vi "Motor-Maker-Triangle RD.vi"() -> ()   [LabVIEW 2021]
panel:
  in  "X Volta":dbl
  out "Motor X\nLigado volt 3":bool=TRUE
  in  "Subida X Descida Y n vezes":i32
  out "Motor Y\nLigado ida 2":bool=TRUE
  in  "Y Descida 2":dbl
  out "Motor X\nLigado ida 2":bool=TRUE
  in  "Xsubida 2":dbl
  in  "SubidaXY em numero par":i32
  in  "Ysubida":dbl
  out "Motor Y\nLigado ida":bool=TRUE
  in  "Xsubida":dbl
  out "Motor X\nLigado ida":bool=TRUE
  # "numero do for loop"
  # "numero do for loop"
  # "N. do motor"
  # "N. do motor"
  # "N. da volta do x"
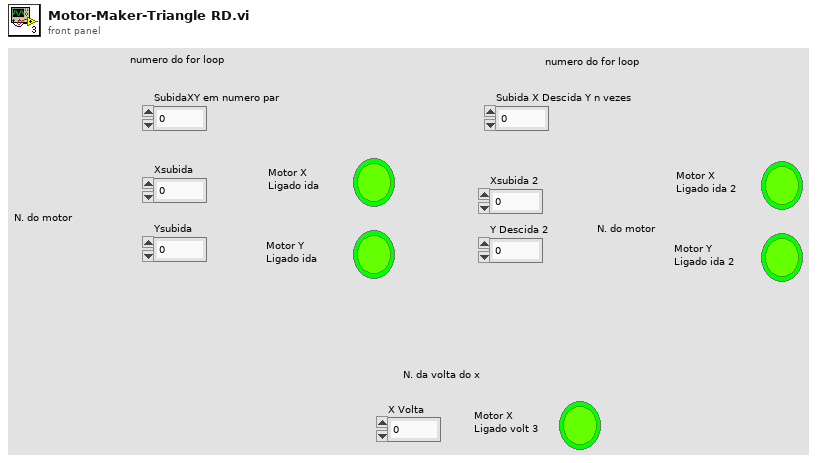
[diagram p1: front panel]
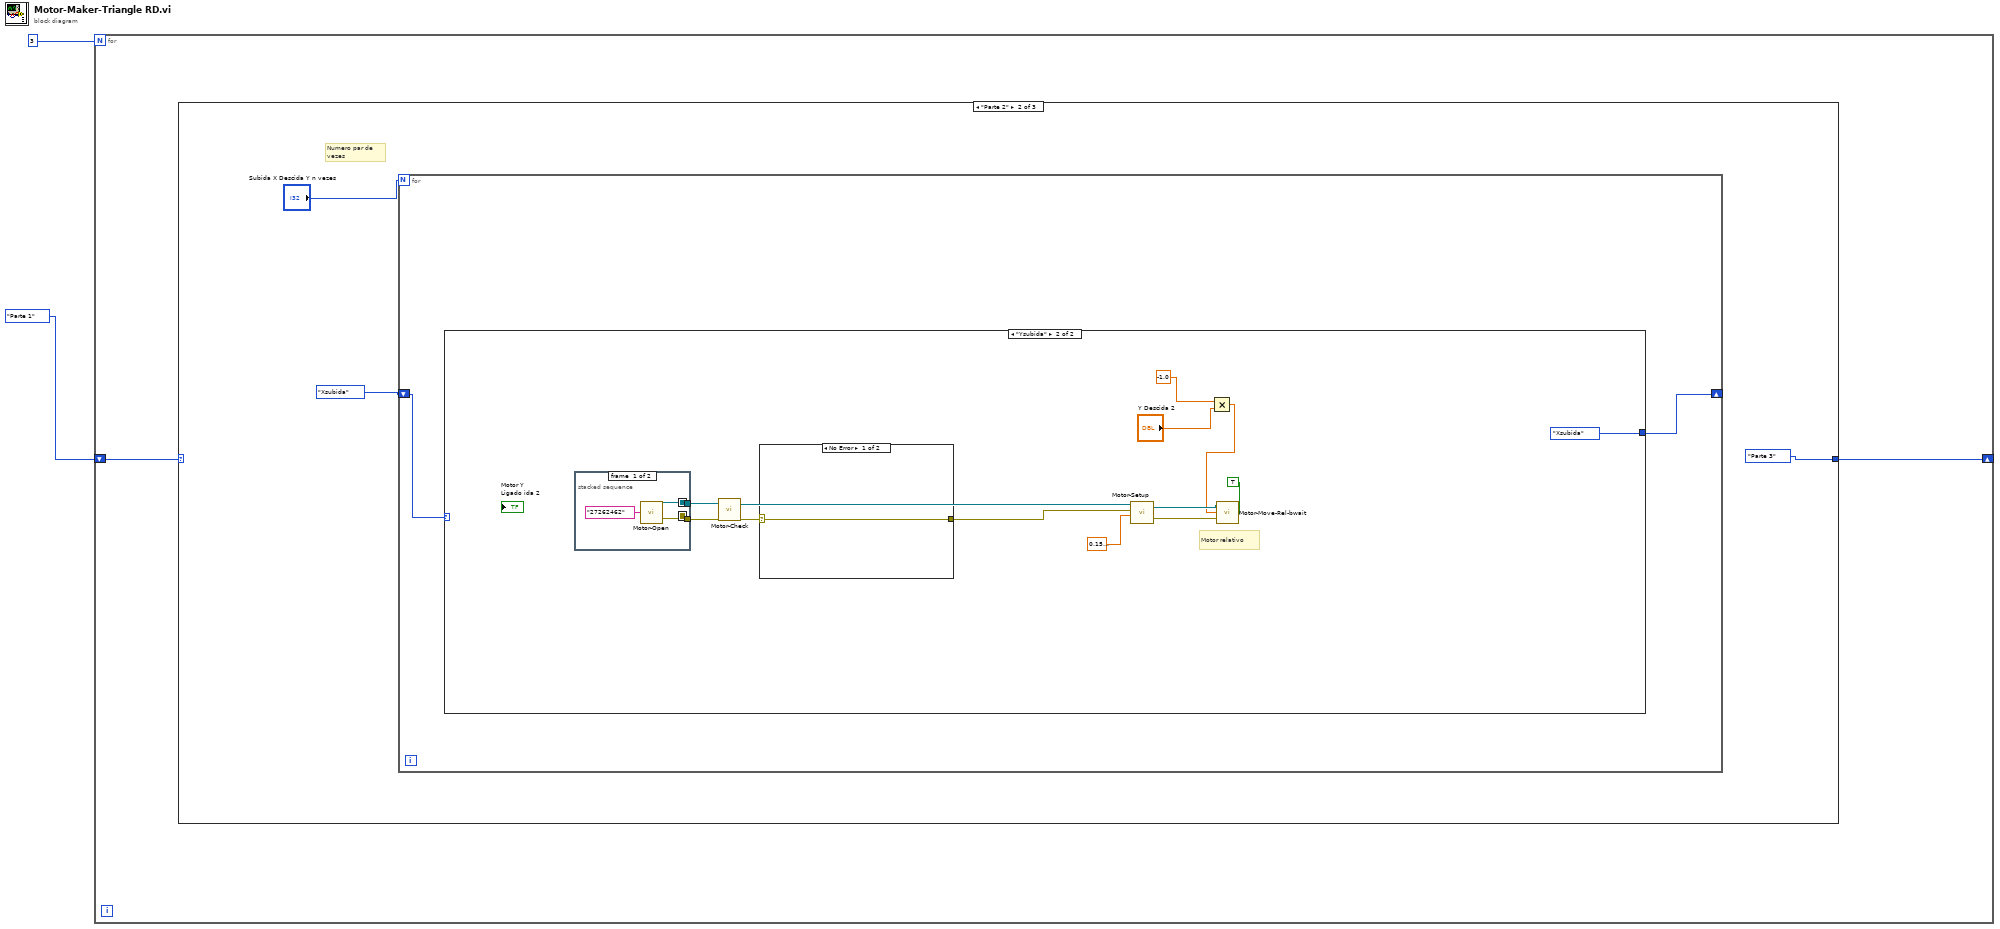
[diagram p0: block diagram]
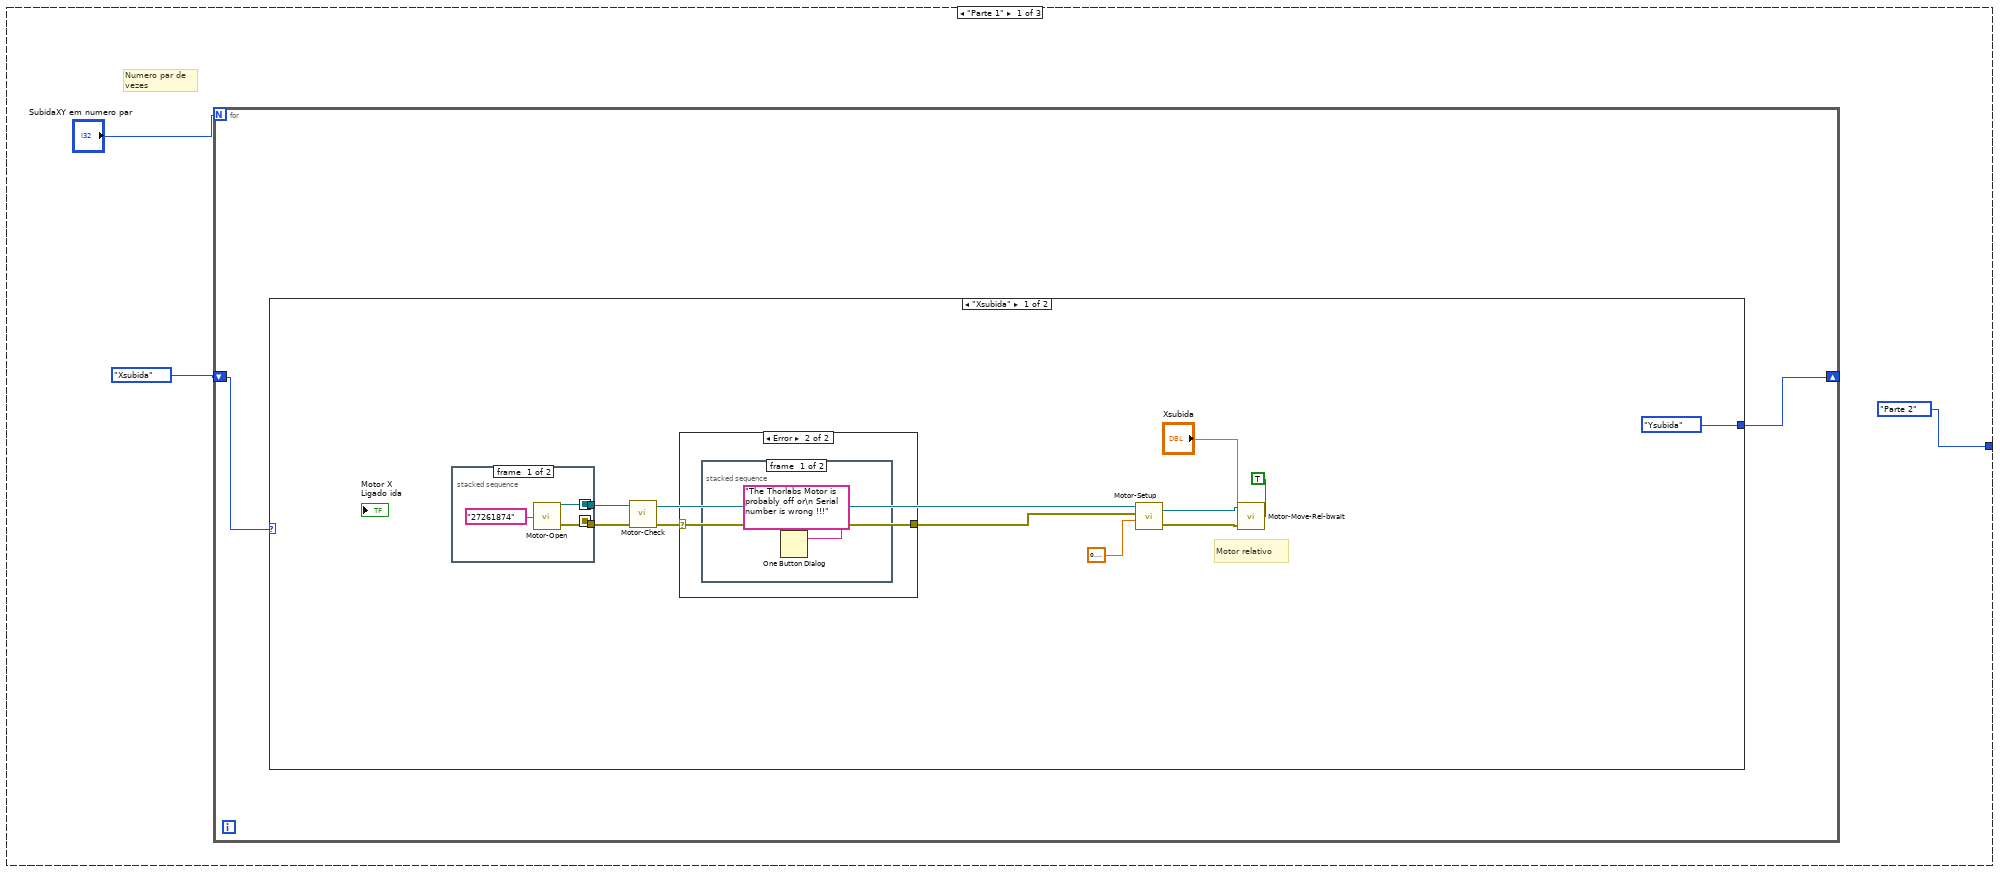
[diagram p2: hidden frame]
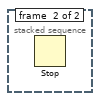
[diagram p4: hidden frame]
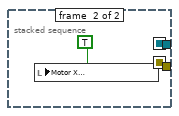
[diagram p5: hidden frame]
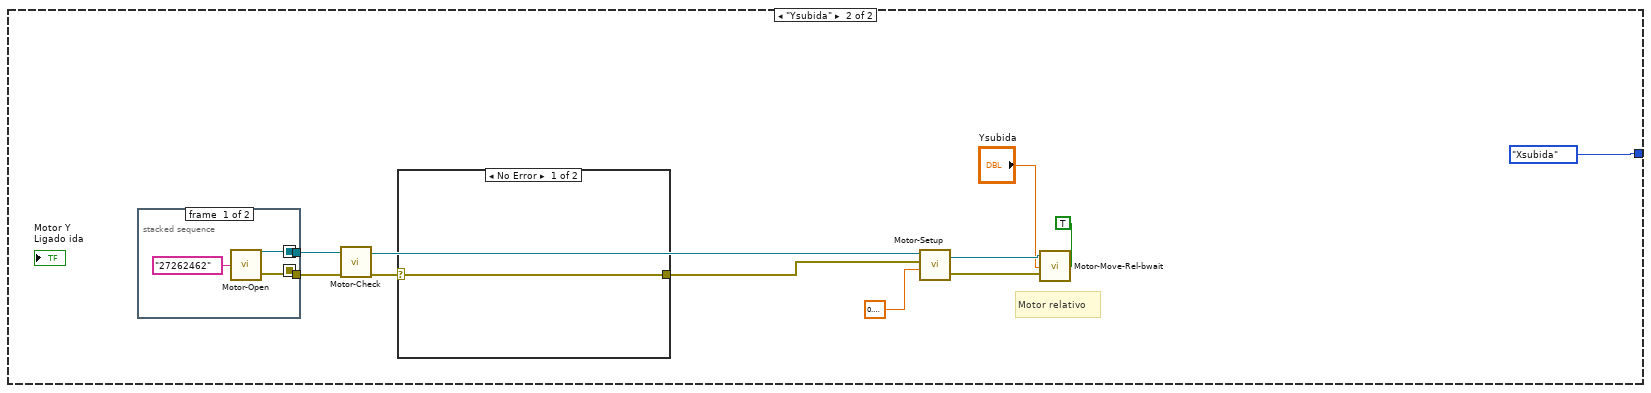
[diagram p6: hidden frame]
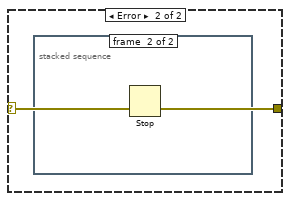
[diagram p7: hidden frame]
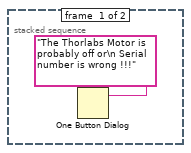
[diagram p8: hidden frame]
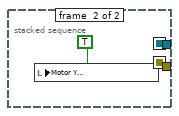
[diagram p9: hidden frame]
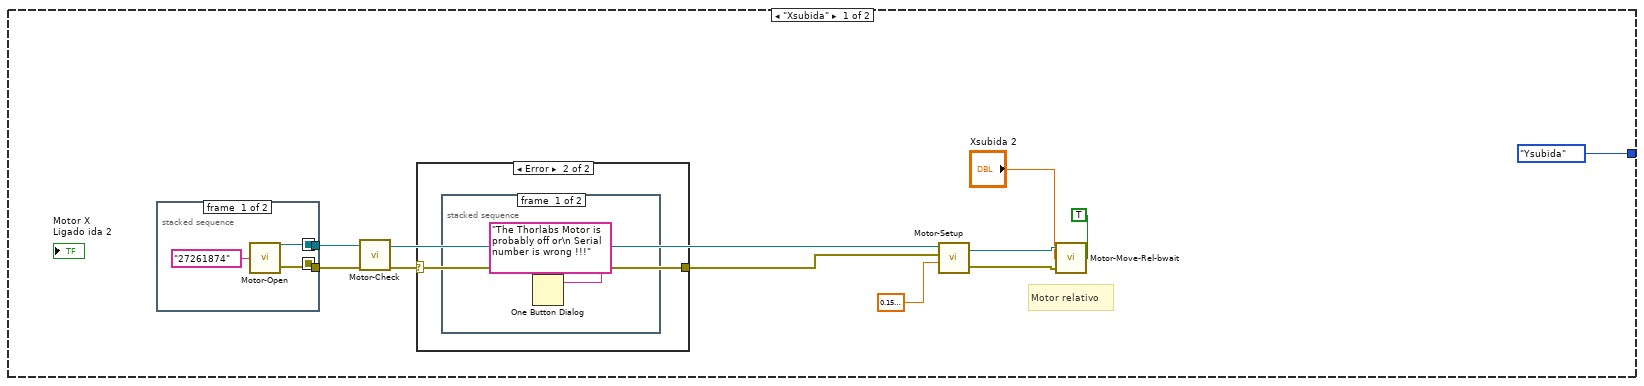
[diagram p10: hidden frame]
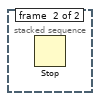
[diagram p12: hidden frame]
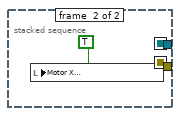
[diagram p13: hidden frame]
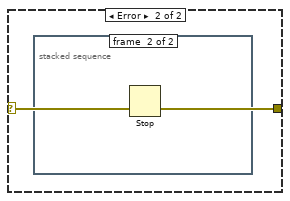
[diagram p14: hidden frame]
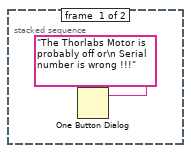
[diagram p15: hidden frame]
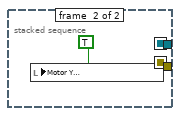
[diagram p16: hidden frame]
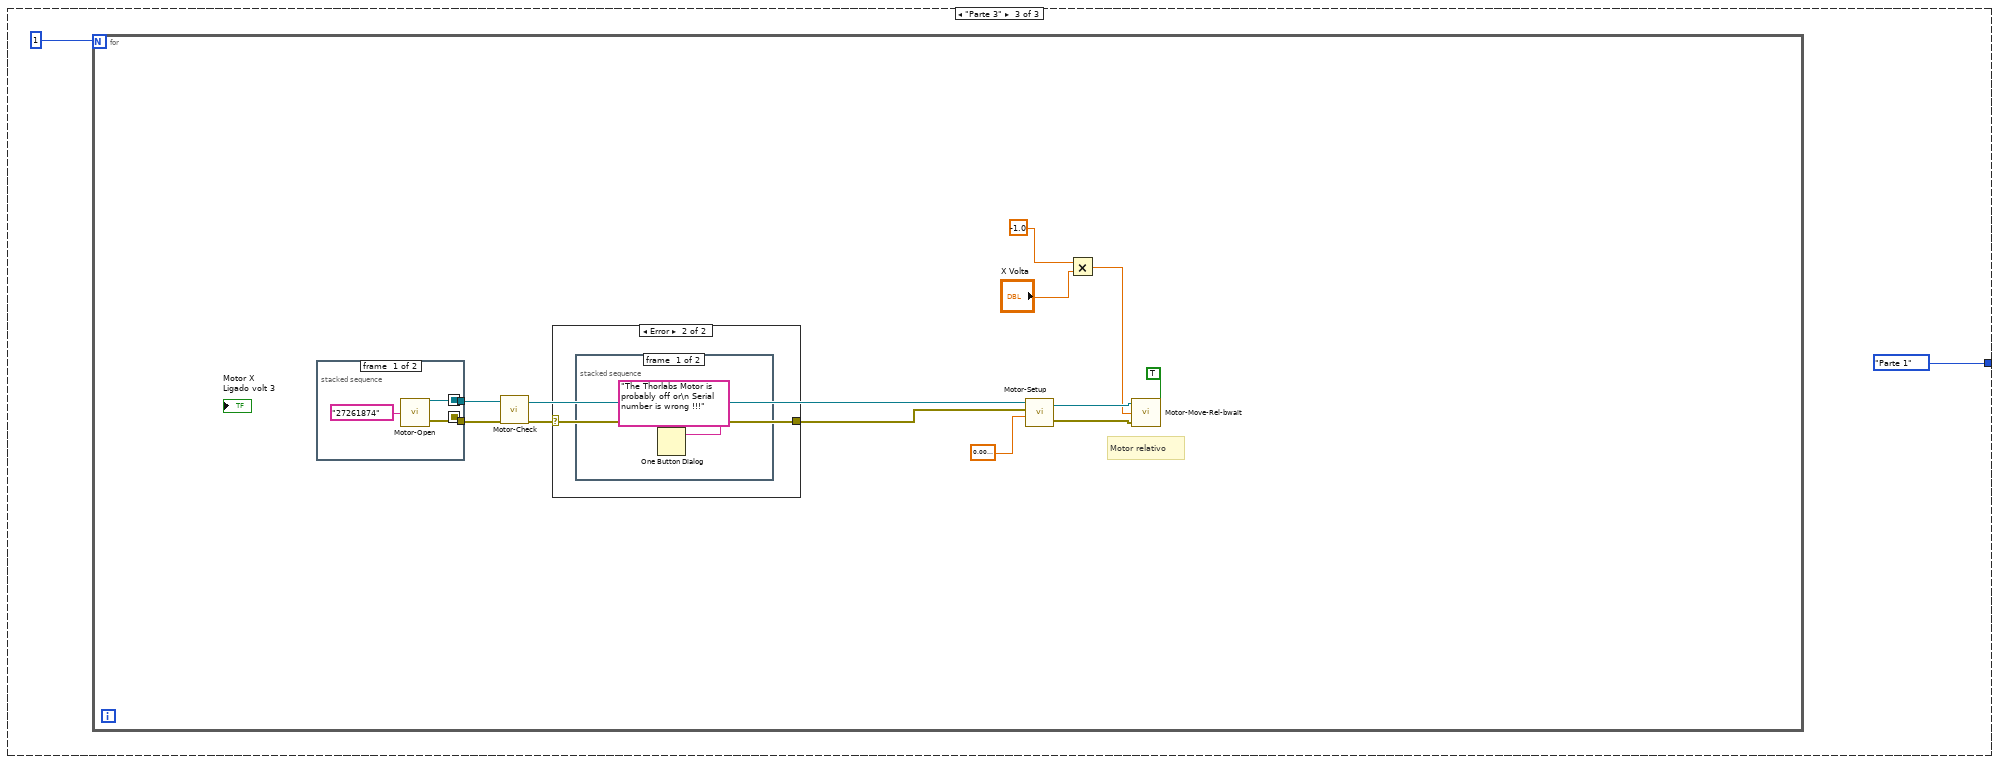
[diagram p17: hidden frame]
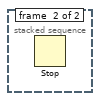
[diagram p19: hidden frame]
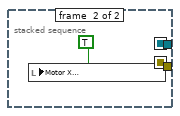
[diagram p20: hidden frame]
diagram:
  n1 = for {
    N: 3 -> [_]
    shift-right: [w3] -> _
    shift-left: enum16{"Parte 1", "Parte 2", "Parte 3"}."Parte 1" -> [w4]
    n2 = case shown="\"Parte 2\"" w4 {
      tunnel: [enum16{"Parte 1", "Parte 2", "Parte 3"}."Parte 2" enum16{"Parte 1", "Parte 2", "Parte 3"}."Parte 3" enum16{"Parte 1", "Parte 2", "Parte 3"}."Parte 1"] -> w3
      frame "Parte 1" {
        # "Numero par de vezes"
        n3 = for {
          N: "SubidaXY em numero par" -> [_]
          shift-right: [w8] -> _
          shift-left: enum16{"Xsubida", "Ysubida"}."Xsubida" -> [w9]
          n4 = case shown="\"Xsubida\"" w9 {
            tunnel: [enum16{"Xsubida", "Ysubida"}."Ysubida" enum16{"Xsubida", "Ysubida"}."Xsubida"] -> w8
            frame "Xsubida" {
              # "Motor relativo"
              n5 = stacked-sequence {
                seq-local: [w26 _] -> [_ w29]
                seq-local: [w25 _] -> [_ w28]
                tunnel: [_ w29] -> w20
                tunnel: [_ w28] -> w19
                frame #0 {
                  n6 = call "Motor-Open.vi"("S/N Motor"="27261874") -> ("MG17Motor 2"=w26:refnum<k7>, "error out"=w25:errorcluster)
                }
                frame #1 {
                  n7 = local write "Motor X\nLigado ida"(TRUE ("Motor3\nLigado")) -> ()
                }
              }
              n8 = call "Motor-Check.vi"("error in (no error)"=w19, "Automation Refnum in"=w20) -> ("error out"=w18:errorcluster, "Automation Refnum out"=w17:refnum<k7>)  [unwired: 8 in]
              n9 = case shown="Error" w18 {
                selector: w18 -> [w21 w22]
                tunnel: [w21 w22] -> w16
                frame No Error {
                }
                frame Error {
                  n10 = stacked-sequence {
                    frame #0 {
                      n11 = One Button Dialog(message="The Thorlabs Motor is probably off or\n Serial number is wrong !!!") -> ()  [unwired: 1 in, 1 out]
                    }
                    frame #1 {
                      n12 = Stop() -> ()  [unwired: 1 in]
                    }
                  }
                }
              }
              n13 = call "Motor-Setup.vi"("Velocidade"=sgl 0.1, "error"=w16, "MG17Motor A"=w17) -> ("error out"=w11:errorcluster, "MG17Motor out"=w12:refnum<k7>)  [unwired: 1 in]
              n14 = call "Motor-Move-Rel-bwait.vi"("bWait"=TRUE, "error"=w11, "Posição"="Xsubida", "MG17Motor A"=w12) -> ()  [unwired: 2 out]
            }
            frame "Ysubida" {
              # "Motor relativo"
              n15 = stacked-sequence {
                seq-local: [w46 _] -> [_ w49]
                seq-local: [w45 _] -> [_ w48]
                tunnel: [_ w49] -> w40
                tunnel: [_ w48] -> w39
                frame #0 {
                  n16 = call "Motor-Open.vi"("S/N Motor"="27262462") -> ("MG17Motor 2"=w46:refnum<k7>, "error out"=w45:errorcluster)
                }
                frame #1 {
                  n17 = local write "Motor Y\nLigado ida"(TRUE ("Motor3\nLigado")) -> ()
                }
              }
              n18 = call "Motor-Check.vi"("error in (no error)"=w39, "Automation Refnum in"=w40) -> ("error out"=w38:errorcluster, "Automation Refnum out"=w37:refnum<k7>)  [unwired: 8 in]
              n19 = case shown="No Error" w38 {
                selector: w38 -> [w41 w42]
                tunnel: [w41 w42] -> w36
                frame No Error {
                }
                frame Error {
                  n20 = stacked-sequence {
                    frame #0 {
                      n21 = One Button Dialog(message="The Thorlabs Motor is probably off or\n Serial number is wrong !!!") -> ()  [unwired: 1 in, 1 out]
                    }
                    frame #1 {
                      n22 = Stop() -> ()  [unwired: 1 in]
                    }
                  }
                }
              }
              n23 = call "Motor-Setup.vi"("Velocidade"=sgl 0.1, "error"=w36, "MG17Motor A"=w37) -> ("error out"=w33:errorcluster, "MG17Motor out"=w34:refnum<k7>)  [unwired: 1 in]
              n24 = call "Motor-Move-Rel-bwait.vi"("bWait"=TRUE, "error"=w33, "Posição"="Ysubida", "MG17Motor A"=w34) -> ()  [unwired: 2 out]
            }
          }
        }
      }
      frame "Parte 2" {
        # "Numero par de vezes"
        n25 = for {
          N: "Subida X Descida Y n vezes" -> [_]
          shift-right: [w53] -> _
          shift-left: enum16{"Xsubida", "Ysubida"}."Xsubida" -> [w54]
          n26 = case shown="\"Ysubida\"" w54 {
            tunnel: [enum16{"Xsubida", "Ysubida"}."Ysubida" enum16{"Xsubida", "Ysubida"}."Xsubida"] -> w53
            frame "Xsubida" {
              # "Motor relativo"
              n27 = stacked-sequence {
                seq-local: [w71 _] -> [_ w74]
                seq-local: [w70 _] -> [_ w73]
                tunnel: [_ w74] -> w65
                tunnel: [_ w73] -> w64
                frame #0 {
                  n28 = call "Motor-Open.vi"("S/N Motor"="27261874") -> ("MG17Motor 2"=w71:refnum<k7>, "error out"=w70:errorcluster)
                }
                frame #1 {
                  n29 = local write "Motor X\nLigado ida 2"(TRUE ("Motor3\nLigado")) -> ()
                }
              }
              n30 = call "Motor-Check.vi"("error in (no error)"=w64, "Automation Refnum in"=w65) -> ("error out"=w63:errorcluster, "Automation Refnum out"=w62:refnum<k7>)  [unwired: 8 in]
              n31 = case shown="Error" w63 {
                selector: w63 -> [w66 w67]
                tunnel: [w66 w67] -> w61
                frame No Error {
                }
                frame Error {
                  n32 = stacked-sequence {
                    frame #0 {
                      n33 = One Button Dialog(message="The Thorlabs Motor is probably off or\n Serial number is wrong !!!") -> ()  [unwired: 1 in, 1 out]
                    }
                    frame #1 {
                      n34 = Stop() -> ()  [unwired: 1 in]
                    }
                  }
                }
              }
              n35 = call "Motor-Setup.vi"("Velocidade"=sgl 0.15, "error"=w61, "MG17Motor A"=w62) -> ("error out"=w56:errorcluster, "MG17Motor out"=w57:refnum<k7>)  [unwired: 1 in]
              n36 = call "Motor-Move-Rel-bwait.vi"("bWait"=TRUE, "error"=w56, "Posição"="Xsubida 2", "MG17Motor A"=w57) -> ()  [unwired: 2 out]
            }
            frame "Ysubida" {
              # "Motor relativo"
              n37 = stacked-sequence {
                seq-local: [w93 _] -> [_ w96]
                seq-local: [w92 _] -> [_ w95]
                tunnel: [_ w96] -> w87
                tunnel: [_ w95] -> w86
                frame #0 {
                  n38 = call "Motor-Open.vi"("S/N Motor"="27262462") -> ("MG17Motor 2"=w93:refnum<k7>, "error out"=w92:errorcluster)
                }
                frame #1 {
                  n39 = local write "Motor Y\nLigado ida 2"(TRUE ("Motor3\nLigado")) -> ()
                }
              }
              n40 = call "Motor-Check.vi"("error in (no error)"=w86, "Automation Refnum in"=w87) -> ("error out"=w85:errorcluster, "Automation Refnum out"=w84:refnum<k7>)  [unwired: 8 in]
              n41 = case shown="No Error" w85 {
                selector: w85 -> [w88 w89]
                tunnel: [w88 w89] -> w83
                frame No Error {
                }
                frame Error {
                  n42 = stacked-sequence {
                    frame #0 {
                      n43 = One Button Dialog(message="The Thorlabs Motor is probably off or\n Serial number is wrong !!!") -> ()  [unwired: 1 in, 1 out]
                    }
                    frame #1 {
                      n44 = Stop() -> ()  [unwired: 1 in]
                    }
                  }
                }
              }
              n45 = call "Motor-Setup.vi"("Velocidade"=sgl 0.15, "error"=w83, "MG17Motor A"=w84) -> ("error out"=w80:errorcluster, "MG17Motor out"=w81:refnum<k7>)  [unwired: 1 in]
              n46 = Multiply(x=-1.0, y="Y Descida 2") -> (x*y=w75:dbl)
              n47 = call "Motor-Move-Rel-bwait.vi"("bWait"=TRUE, "error"=w80, "Posição"=w75, "MG17Motor A"=w81) -> ()  [unwired: 2 out]
            }
          }
        }
      }
      frame "Parte 3" {
        n48 = for {
          N: 1 -> [_]
          # "Motor relativo"
          n49 = stacked-sequence {
            seq-local: [w116 _] -> [_ w119]
            seq-local: [w115 _] -> [_ w118]
            tunnel: [_ w119] -> w110
            tunnel: [_ w118] -> w109
            frame #0 {
              n50 = call "Motor-Open.vi"("S/N Motor"="27261874") -> ("MG17Motor 2"=w116:refnum<k7>, "error out"=w115:errorcluster)
            }
            frame #1 {
              n51 = local write "Motor X\nLigado volt 3"(TRUE ("Motor3\nLigado")) -> ()
            }
          }
          n52 = call "Motor-Check.vi"("error in (no error)"=w109, "Automation Refnum in"=w110) -> ("error out"=w108:errorcluster, "Automation Refnum out"=w107:refnum<k7>)  [unwired: 8 in]
          n53 = case shown="Error" w108 {
            selector: w108 -> [w111 w112]
            tunnel: [w111 w112] -> w106
            frame No Error {
            }
            frame Error {
              n54 = stacked-sequence {
                frame #0 {
                  n55 = One Button Dialog(message="The Thorlabs Motor is probably off or\n Serial number is wrong !!!") -> ()  [unwired: 1 in, 1 out]
                }
                frame #1 {
                  n56 = Stop() -> ()  [unwired: 1 in]
                }
              }
            }
          }
          n57 = call "Motor-Setup.vi"("Velocidade"=sgl 0.01, "error"=w106, "MG17Motor A"=w107) -> ("error out"=w102:errorcluster, "MG17Motor out"=w103:refnum<k7>)  [unwired: 1 in]
          n58 = Multiply(x=-1.0, y="X Volta") -> (x*y=w99:dbl)
          n59 = call "Motor-Move-Rel-bwait.vi"("bWait"=TRUE, "error"=w102, "Posição"=w99, "MG17Motor A"=w103) -> ()  [unwired: 2 out]
        }
      }
    }
  }
